vi "2-4040_Set SampleNumber&AcquireData.vi"(6 "Start/Stop 2":refnum<vi>, 8 "error in (no error)":errorcluster, 9 "WaveForm(3)":refnum<vi>[](array[refnum]), 10 "Sample Number":i32, 11 "VISA resource name":refnum<visa-resource-name>) -> (0 "error out":errorcluster, 1 "Pressure":dbl[](array[numeric]), 2 "Tem":dbl[](array[numeric]), 3 "Flow":dbl[](array[numeric]))   [LabVIEW 2017]
uses:
  <vilib>/Instr/_visa.llb/VISA Flush IO Buffer Mask.ctl
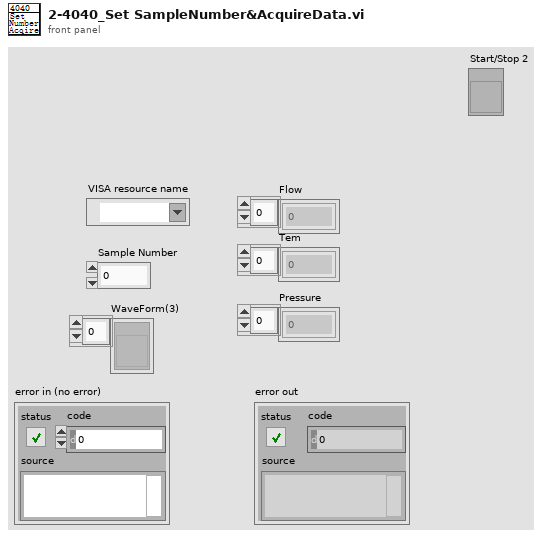
[diagram p1: front panel]
types:
  T1 = typedef "VISA Flush IO Buffer Mask.ctl" = u16
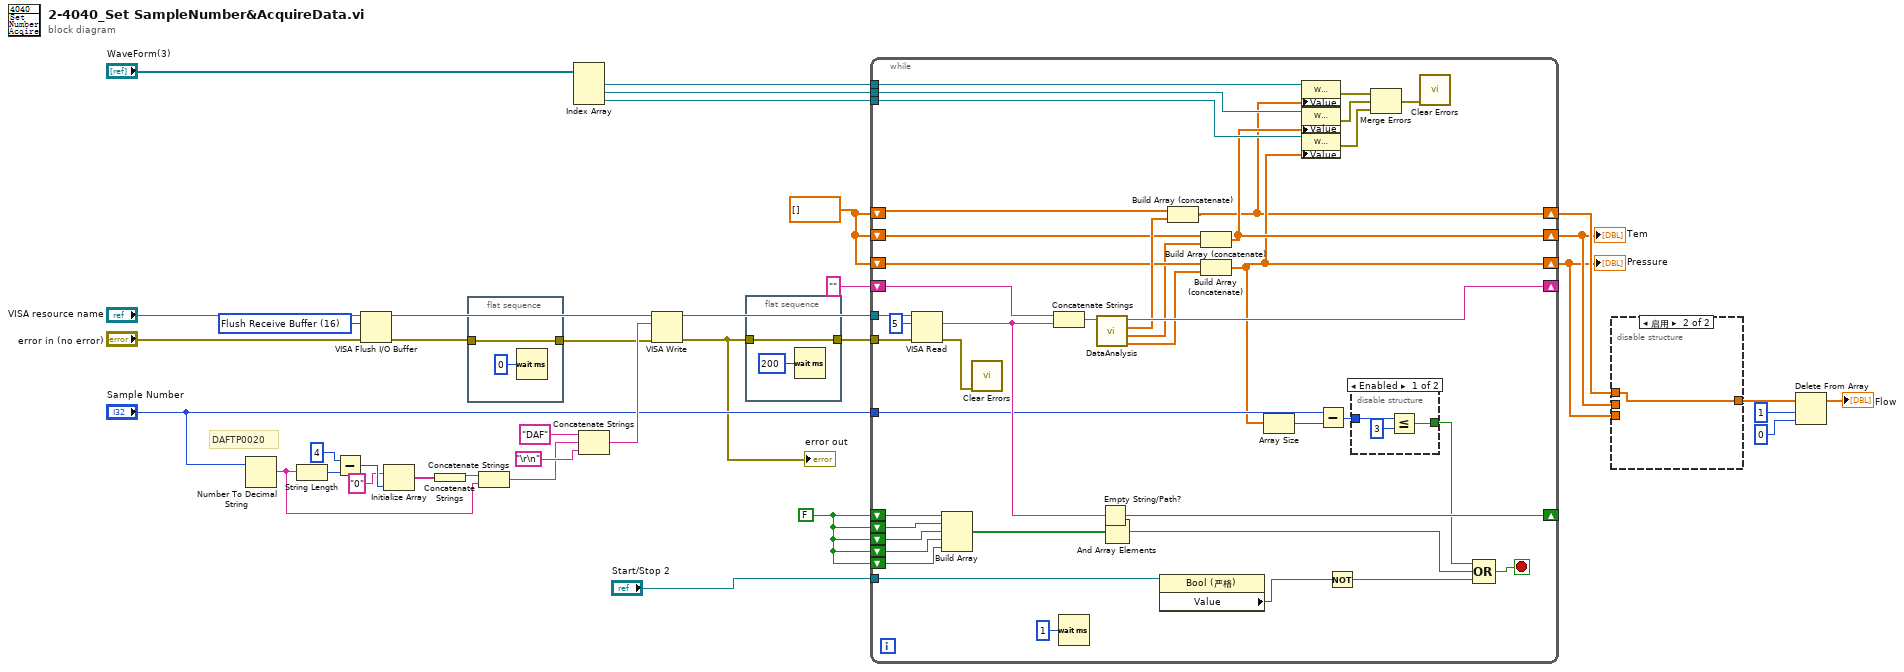
[diagram p0: block diagram]
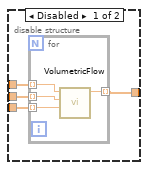
[diagram p2: hidden frame]
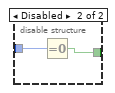
[diagram p3: hidden frame]
diagram:
  w12 = T1 16 items=["Flush Receive Buffer"=16, "Write Transmit Buffer to Device"=32, "Flush Receive Buffer (No I/O)"=64, "Flush Transmit Buffer"=128] ("Mask")
  w16 = dbl[] []
  w19 = FALSE
  # "DAFTP0020"
  n1 = Number To Decimal String(number="Sample Number") -> (decimal integer string=w28:string)  [unwired: 1 in]
  n2 = String Length(string=w28) -> (length=w34:i32)
  n3 = Subtract(x=4, y=w34) -> (x-y=w32:i32)
  n4 = VISA Flush I/O Buffer(VISA resource name="VISA resource name", mask (16)=w12, error in (no error)="error in (no error)") -> (VISA resource name out=w14:refnum<visa-resource-name>, error out=w11:errorcluster)
  n5 = Initialize Array("0", w32) -> (w30:string[])
  n6 = Concatenate Strings(w30) -> (w29:string)
  n7 = flat-sequence {
    tunnel: w11 -> [w38]
    tunnel: [w38] -> w10
    frame #0 {
      n8 = Wait (ms)(milliseconds to wait=u32 0) -> ()  [unwired: 1 out]
    }
  }
  n9 = Concatenate Strings(w29, w28) -> (w27:string)
  n10 = Index Array(array="WaveForm(3)") -> (element #1=w22:refnum<vi>, element #2=w21:refnum<vi>, element #3=w20:refnum<vi>)  [unwired: 3 in]
  n11 = Concatenate Strings("DAF" ("写入缓冲区"), w27, "\r\n") -> (w26:string)
  n12 = VISA Write(VISA resource name=w14, write buffer=w26, error in (no error)=w10) -> (VISA resource name out=w25:refnum<visa-resource-name>, error out=w9:errorcluster)  [unwired: 1 out]
  "error out" <- w9
  n13 = flat-sequence {
    tunnel: w9 -> [w40]
    tunnel: [w40] -> w17
    frame #0 {
      n14 = Wait (ms)(milliseconds to wait=u32 200) -> ()  [unwired: 1 out]
    }
  }
  n15 = while {
    tunnel: w17 -> [w80]
    tunnel: w25 -> [w81]
    shift-right: [w73] -> _
    shift-left: "" -> [w75]
    tunnel: w22 -> [w78]
    tunnel: w21 -> [w76]
    tunnel: w20 -> [w77]
    shift-right: [w70] -> _
    shift-left: w19 -> [w69]
    shift-left: w19 -> [w68]
    shift-left: w19 -> [w67]
    shift-left: w19 -> [w66]
    shift-left: w19 -> [w65]
    tunnel: "Sample Number" -> [w61]
    shift-right: [w44] -> w8
    shift-left: w16 -> [w58]
    shift-right: [w46] -> w7
    shift-left: w16 -> [w56]
    shift-right: [w45] -> w6
    shift-left: w16 -> [w55]
    tunnel: "Start/Stop 2" -> [w43]
    stop <- w60 stop-if-true
    n16 = VISA Read(VISA resource name=w81, byte count=u32 5 ("字节总数"), error in (no error)=w80) -> (read buffer=w71:string, error out=w72:errorcluster)  [unwired: 2 out]
    n17 = Build Array(w69, w68, w67, w66, w65) -> (w64:bool[])
    n18 = call <vilib>:"Clear Errors.vi"("error in (no error)"=w72) -> ()  [unwired: 5 in, 2 out]
    n19 = Concatenate Strings(w75, w71) -> (w74:string)
    n20 = Wait (ms)(milliseconds to wait=u32 1) -> ()  [unwired: 1 out]
    n21 = call "DataAnalysis.vi"("Data"=w74) -> ("3"=w53:dbl[], "2"=w54:dbl[], "1"=w57:dbl[], "Residue Datas"=w73:string)  [unwired: 6 in, 1 out]
    n22 = Empty String/Path?(string/path=w71) -> (empty?=w70:bool)
    n23 = And Array Elements(Boolean array=w64) -> (logical AND=w63:bool)
    n24 = property class="Bool (严格)"(reference=w43) -> ("Value"=w42:bool)  [unwired: 1 in, 2 out]
    n25 = Build Array (concatenate)(w58, w57) -> (w44:dbl[])
    n26 = Build Array (concatenate)(w56, w54) -> (w46:dbl[])
    n27 = Build Array (concatenate)(w55, w53) -> (w45:dbl[])
    n28 = Array Size(array=w45) -> (size(s)=w48:i32)
    n29 = property class="WFGraph (strict)"(reference=w78, "Value"=w44) -> (error out=w52:errorcluster)  [unwired: 1 in, 1 out]
    n30 = property class="WFGraph (strict)"(reference=w76, "Value"=w46) -> (error out=w51:errorcluster)  [unwired: 1 in, 1 out]
    n31 = property class="WFGraph (strict)"(reference=w77, "Value"=w45) -> (error out=w50:errorcluster)  [unwired: 1 in, 1 out]
    n32 = Subtract(x=w61, y=w48) -> (x-y=w62:i32)
    n33 = Not(x=w42) -> (.not. x?=w41:bool)
    n34 = disable-structure shown="Enabled" {
      disable-tunnel: w62 -> [w84 w85]
      disable-tunnel: [w82 w86] -> w59
      frame Enabled {
        n35 = Less Or Equal?(x=w84, y=3) -> (x <= y?=w82:bool)
      }
      frame Disabled {
        n36 = Equal To 0?(x=w85) -> (x = 0?=w86:bool)
      }
    }
    n37 = Merge Errors(w52, w51, w50) -> (w49:errorcluster)
    n38 = call <vilib>:"Clear Errors.vi"("error in (no error)"=w49) -> ()  [unwired: 5 in, 2 out]
    n39 = Compound Arithmetic op=OR(w59, w63, w41) -> (w60:bool)
  }
  "Tem" <- w7
  "Pressure" <- w6
  n40 = disable-structure shown="启用" {
    disable-tunnel: w8 -> [w90 w95]
    disable-tunnel: w7 -> [w89 _]
    disable-tunnel: w6 -> [w88 _]
    disable-tunnel: [w87 w95] -> w5
    frame Disabled {
      n41 = for {
        tunnel: w90 -> [w94] mode=indexing
        tunnel: w89 -> [w93] mode=indexing
        tunnel: w88 -> [w92] mode=indexing
        tunnel: [w91] -> w87 mode=indexing
        n42 = call "VolumetricFlow.vi"("Pressure"=w92, "Tem"=w93, "Flow"=w94) -> ("VolumetricFlow"=w91:dbl)  [unwired: 8 in]
      }
    }
    frame Enabled {
    }
  }
  n43 = Delete From Array ("删除数组元素")(array=w5, length=1 ("长度"), index=0 ("索引")) -> (array with subset deleted=→"Flow":dbl[])  [unwired: 1 out]
